vi "CfgFile Set Desc i.vi"(8 "error in (no error)":errorcluster, 10 "i":T1, 11 "LF2R IDE in":refnum<class "LF2R IDE.lvclass">) -> (0 "error out":errorcluster, 3 "LF2R IDE out":refnum<class "LF2R IDE.lvclass">)   [LabVIEW 2018, in "LF2R IDE.lvlib" / "LF2R IDE.lvclass"]
uses:
  LF2R IDE.lvclass
  Const UI Desc Frame i.ctl
  Const UI Desc Property.ctl
  LF2R IDE.lvclass/LF2R IDE.ctl
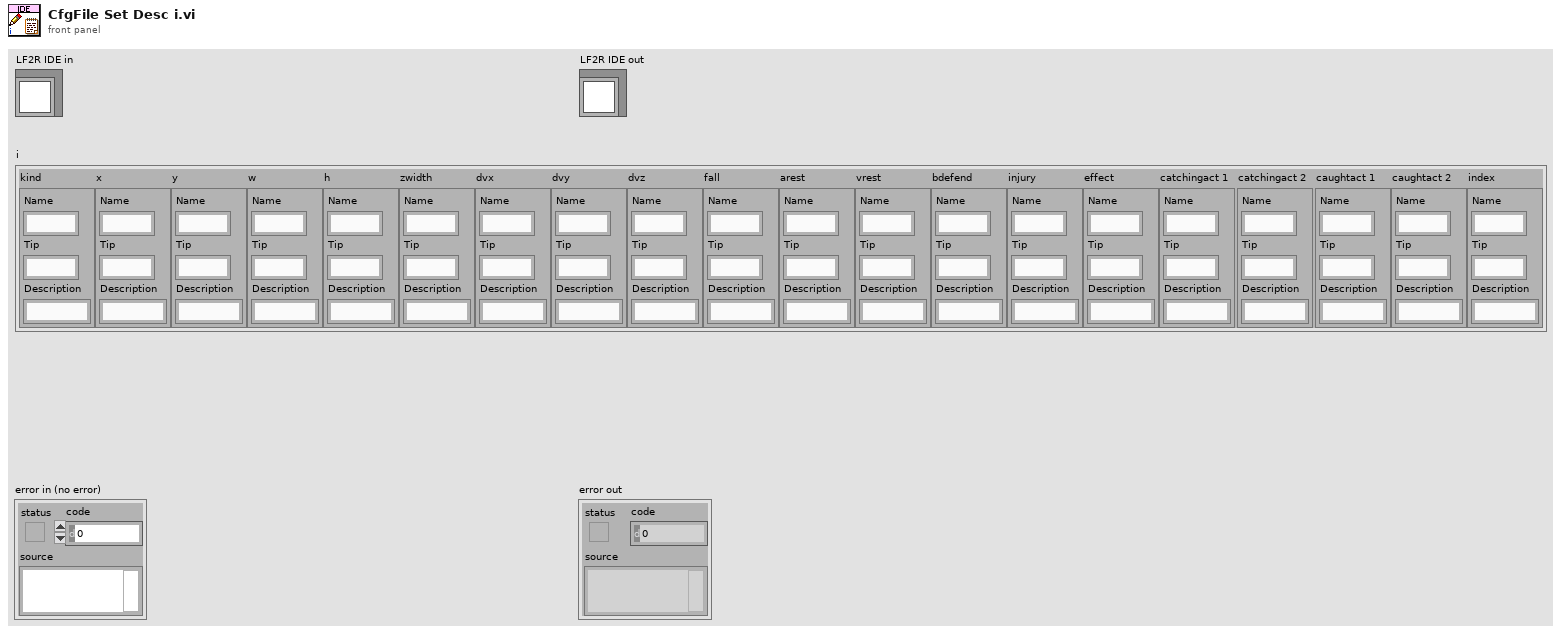
[diagram p1: front panel]
types:
  T1 = typedef "LF2R IDE.lvlib/LF2R IDE.lvclass/Const UI Desc Frame i.ctl" = cluster{"kind":T2, "x":T2, "y":T2, "w":T2, "h":T2, "zwidth":T2, "dvx":T2, "dvy":T2, "dvz":T2, "fall":T2, "arest":T2, "vrest":T2, "bdefend":T2, "injury":T2, "effect":T2, "catchingact 1":T2, "catchingact 2":T2, "caughtact 1":T2, "caughtact 2":T2, "index":T2}
  T2 = typedef "LF2R IDE.lvlib/LF2R IDE.lvclass/Const UI Desc Property.ctl" = cluster{"Name":string, "Tip":string, "Description":string}
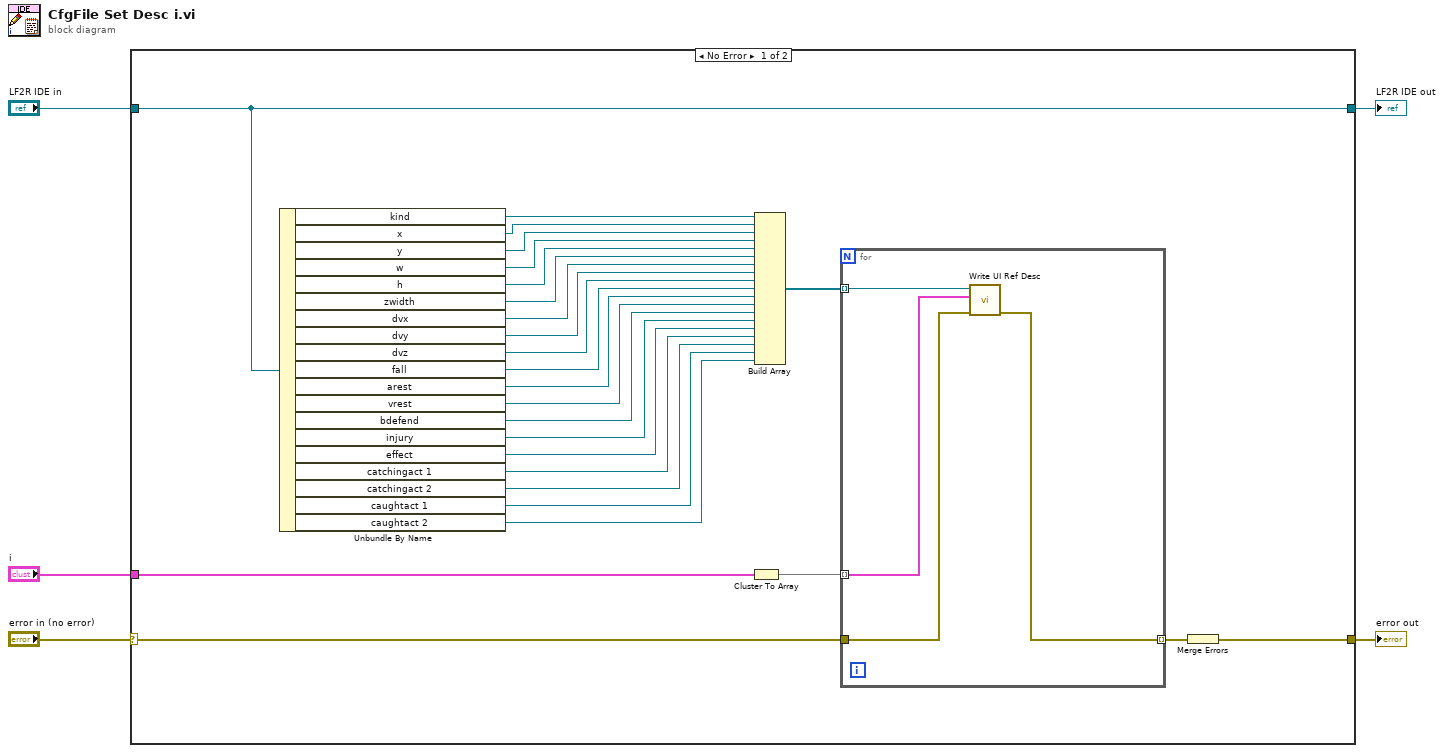
[diagram p0: block diagram]
diagram:
  n1 = case shown="No Error" "error in (no error)" {
    selector: "error in (no error)" -> [w27 w37]
    tunnel: [w25 w37] -> w4
    tunnel: [w31 w36] -> w2
    tunnel: "LF2R IDE in" -> [w31 w36]
    tunnel: "i" -> [w29 _]
    frame No Error {
      n2 = Unbundle By Name(w31) -> ("kind"=w24:refnum<vi>, "x"=w23:refnum<vi>, "y"=w22:refnum<vi>, "w"=w21:refnum<vi>, "h"=w20:refnum<vi>, "zwidth"=w19:refnum<vi>, "dvx"=w18:refnum<vi>, "dvy"=w17:refnum<vi>, "dvz"=w16:refnum<vi>, "fall"=w15:refnum<vi>, "arest"=w14:refnum<vi>, "vrest"=w13:refnum<vi>, "bdefend"=w12:refnum<vi>, "injury"=w11:refnum<vi>, "effect"=w10:refnum<vi>, "catchingact 1"=w9:refnum<vi>, "catchingact 2"=w8:refnum<vi>, "caughtact 1"=w7:refnum<vi>, "caughtact 2"=w6:refnum<vi>)
      n3 = Cluster To Array(cluster=w29) -> (array=w28:T2[])
      n4 = Build Array(w24, w23, w22, w21, w20, w19, w18, w17, w16, w15, w14, w13, w12, w11, w10, w9, w8, w7, w6) -> (w30:refnum<vi>[])
      n5 = for {
        tunnel: w30 -> [w32] mode=indexing
        tunnel: w28 -> [w35] mode=indexing
        tunnel: w27 -> [w34]
        tunnel: [w33] -> w26 mode=indexing
        n6 = call "Write UI Ref Desc.vi"("error in (no error)"=w34, "UI Property"=w35, "UI Ref"=w32) -> ("error out"=w33:errorcluster)  [unwired: 8 in]
      }
      n7 = Merge Errors(w26) -> (w25:errorcluster)
    }
    frame Error {
    }
  }
  "error out" <- w4
  "LF2R IDE out" <- w2
